vi "OAT Timebase Plot.vi"   [LabVIEW 2017]
doc: "Draws a timebase plot on an XY graph. You can use this polymorphic VI with unfiltered or filtered data. The unfiltered data comes from the <B>even angle signals</B> input, the filtered data from the <B>magnitudes</B> and <B>phases [phase lag]</B> inputs. The timebase plot displays the amplitude of a signal as a function of time and marks the tachometer trigger point on the plot. The data type you wire to the <B>even angle signals</B> input determines the polymorphic instance to use."
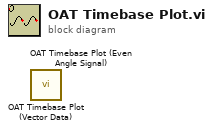
[diagram p0: block diagram]
diagram:
  n1 = call <vilib>:"OAT Timebase Plot (Vector Data).vi"() -> ()  [unwired: 13 in, 3 out]
  n2 = call <vilib>:"OAT Timebase Plot (Even Angle Signal).vi"() -> ()  [unwired: 13 in, 3 out]
